vi "Com_Panel_Panel Return To Default.vi"(8 "error in":errorcluster, 11 "VI Refnum In":refnum<vi>) -> (0 "error out":errorcluster, 3 "VI Refnum Out":refnum<vi>)   [LabVIEW 2016]
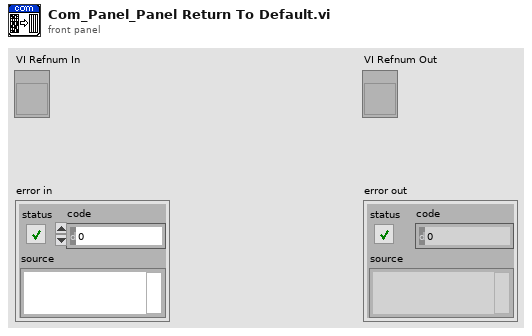
[diagram p1: front panel]
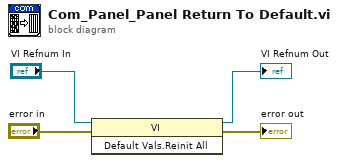
[diagram p0: block diagram]
diagram:
  n1 = invoke class="VI" method="Default Vals.Reinit All"(reference="VI Refnum In", error in="error in") -> (reference out=→"VI Refnum Out":refnum<vi>, error out=→"error out":errorcluster)  [unwired: 1 in, 1 out]
